vi "YAFTAF_Constructor.vi"(8 "ErrorIn":errorcluster, 10 "CmdData":variant, 11 "LocalIn":refnum<class>) -> (0 "ErrorOut":errorcluster, 2 "ReplyData":variant, 3 "LocalIn":refnum<class>, 4 "Exit":bool)   [LabVIEW 2021, in "YAFTAF.lvclass"]
doc: "Used to initialize the attributes of the object. This is called at the creation of the object. This VI can be overridden by the child classes to initialize their attributesa"
uses:
  YAFTAF.lvclass
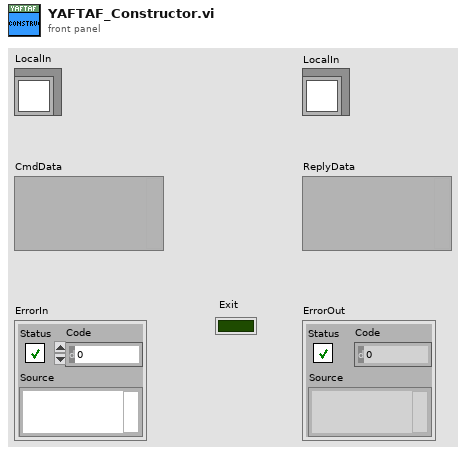
[diagram p1: front panel]
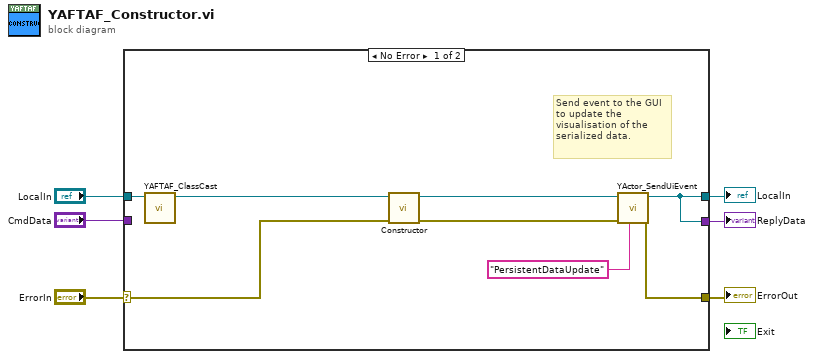
[diagram p0: block diagram]
diagram:
  n1 = case shown="No Error" "ErrorIn" {
    selector: "ErrorIn" -> [w14 w17]
    tunnel: [w13 w17] -> w5
    tunnel: [w10 w16] -> w3
    tunnel: "CmdData" -> [_ w16]
    tunnel: "LocalIn" -> [w11 w15]
    tunnel: [w10 w15] -> w1
    frame No Error {
      # "Send event to the GUI to update the visualisation of the  serialized data."
      n2 = call "YAFTAF_ClassCast.vi"("LocalIn"=w11) -> ("LocalOut"=w8:refnum<class "YAFTAF.lvclass">)  [unwired: 10 in]
      n3 = call-dynamic "Constructor.vi"("ErrorIn"=w14, "ObjectIn"=w8) -> ("ErrorOut"=w12:errorcluster, "ObjectOut"=w7:refnum<class "YAFTAF.lvclass">)  [unwired: 8 in]
      n4 = call-dynamic "YActor_SendUiEvent.vi"("Event"="PersistentDataUpdate", "ErrorIn"=w12, "YActorIn"=w7) -> ("ErrorOut"=w13:errorcluster, "YActorOut"=w10:refnum<class "YAFTAF.lvclass">)  [unwired: 7 in]
    }
    frame Error {
    }
  }
  "ErrorOut" <- w5
  "LocalIn" <- w1
  "ReplyData" <- w3
